vi "Program13.vi"() -> ()   [LabVIEW 2020]
panel:
  out "Waveform Chart 2":i32(graph)
  out "Waveform Chart":i32(graph)
  in  "stop":bool
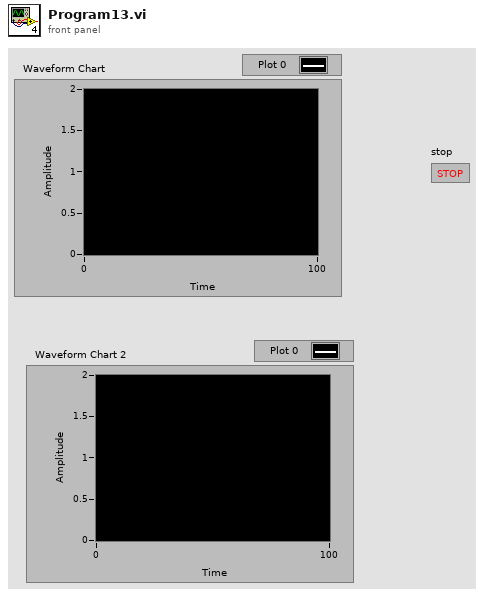
[diagram p1: front panel]
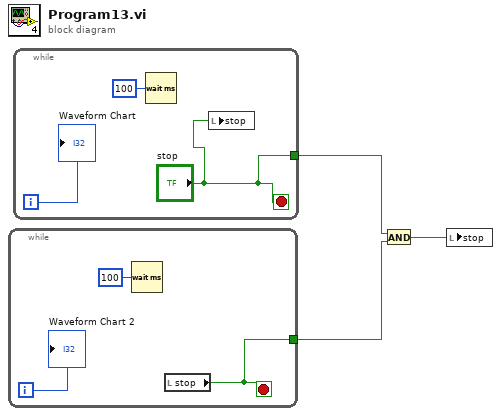
[diagram p0: block diagram]
diagram:
  n1 = while {
    tunnel: [w6] -> w3
    i -> [w5]
    stop <- w6 stop-if-true
    n2 = Wait (ms)(milliseconds to wait=u32 100) -> ()  [unwired: 1 out]
    n3 = local read "stop"() -> (w6:bool)
    "Waveform Chart 2" <- w5
  }
  n4 = while {
    tunnel: ["stop"] -> w2
    i -> [w9]
    stop <- "stop" stop-if-true
    n5 = Wait (ms)(milliseconds to wait=u32 100) -> ()  [unwired: 1 out]
    n6 = local write "stop"("stop") -> ()
    "Waveform Chart" <- w9
  }
  n7 = And(x=w2, y=w3) -> (x .and. y?=w1:bool)
  n8 = local write "stop"(w1) -> ()
